vi "setParameters.vi"(10 "Parameters":T1, 11 "ApplyAOSCorrectionByForcesCommand in":refnum<class "ApplyAOSCorrectionByForcesCommand.lvclass">) -> (3 "ApplyAOSCorrectionByForcesCommand out":refnum<class "ApplyAOSCorrectionByForcesCommand.lvclass">)   [LabVIEW 2016, in "ApplyAOSCorrectionByForcesCommand.lvclass"]
uses:
  ApplyAOSCorrectionByForcesCommand.lvclass
  DataTypes/Topics/CommandApplyAOSCorrectionByForces.ctl
  DataTypes/Topics/Parts/CommandId.ctl
  ApplyAOSCorrectionByForcesCommand.lvclass/ApplyAOSCorrectionByForcesCommand.ctl
  DataTypes/Topics/M1M3SupportTopics.lvlib
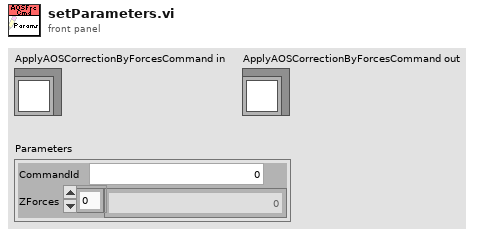
[diagram p1: front panel]
types:
  T1 = typedef "M1M3SupportTopics.lvlib/CommandApplyAOSCorrectionByForces.ctl" = cluster{"CommandId":T2, "ZForces":dbl[]}
  T2 = typedef "M1M3SupportTopics.lvlib/CommandId.ctl" = i32
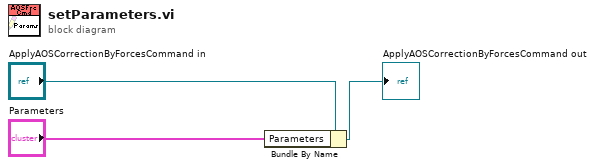
[diagram p0: block diagram]
diagram:
  n1 = Bundle By Name(cluster="ApplyAOSCorrectionByForcesCommand in", "Parameters"="Parameters") -> (→"ApplyAOSCorrectionByForcesCommand out":refnum<class "ApplyAOSCorrectionByForcesCommand.lvclass">)
